vi "video.update_commit.vi"(8 "error in":errorcluster, 11 "VideoUpdateStaging in":refnum<class "VideoUpdateStaging.lvclass">) -> (0 "error out":errorcluster, 3 "VideoUpdateStaging out":refnum<class "VideoUpdateStaging.lvclass">)   [LabVIEW 2020, in "VideoUpdateStaging.lvclass"]
doc: "Applies the staged changes to the video with the given RID and returns a handle to the updated video."
uses:
  VideoUpdateStaging.lvclass
  VideoUpdateStaging.lvclass/VideoUpdateStaging.ctl
  client.lvlib
panel:
  out "out_video out":i32
  in  "rid":string
  in  "staging":i32
  in  "out_video":i32
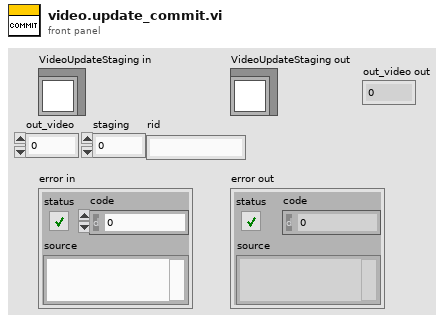
[diagram p1: front panel]
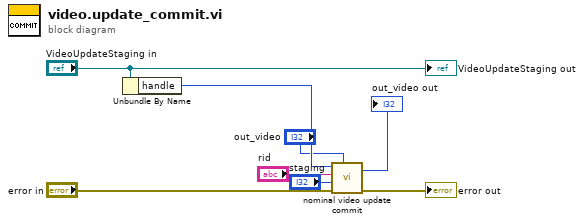
[diagram p0: block diagram]
diagram:
  n1 = Unbundle By Name("VideoUpdateStaging in") -> ("handle"=w6:i32)
  n2 = call "nominal video update commit.vi"("out_video"="out_video", "error in (no error)"="error in", "staging"="staging", "rid"="rid", "client"=w6) -> ("error out"=→"error out":errorcluster, "out_video out"=→"out_video out":i32)  [unwired: 4 in, 1 out]
  "VideoUpdateStaging out" <- "VideoUpdateStaging in"
